vi "writeCounterMasterBatch.vi"(8 "ROI Parameters":T1, 9 "Drop Time (ms)":dbl, 10 "Scan name":string, 11 "file (use dialog)":path) -> ()   [LabVIEW 2015]
uses:
  Controls/ScanParameters/ROI_set.ctl
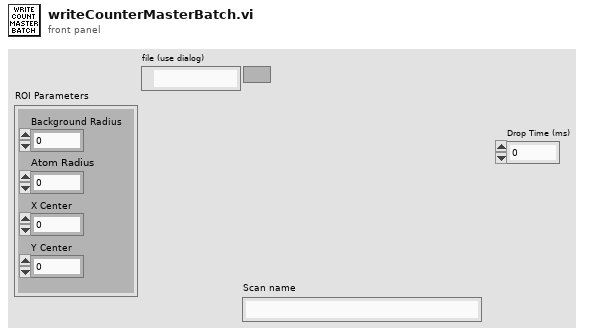
[diagram p1: front panel]
types:
  T1 = typedef "ROI_set.ctl" = cluster{"Background Radius":dbl, "Atom Radius":dbl, "X Center":dbl, "Y Center":dbl}
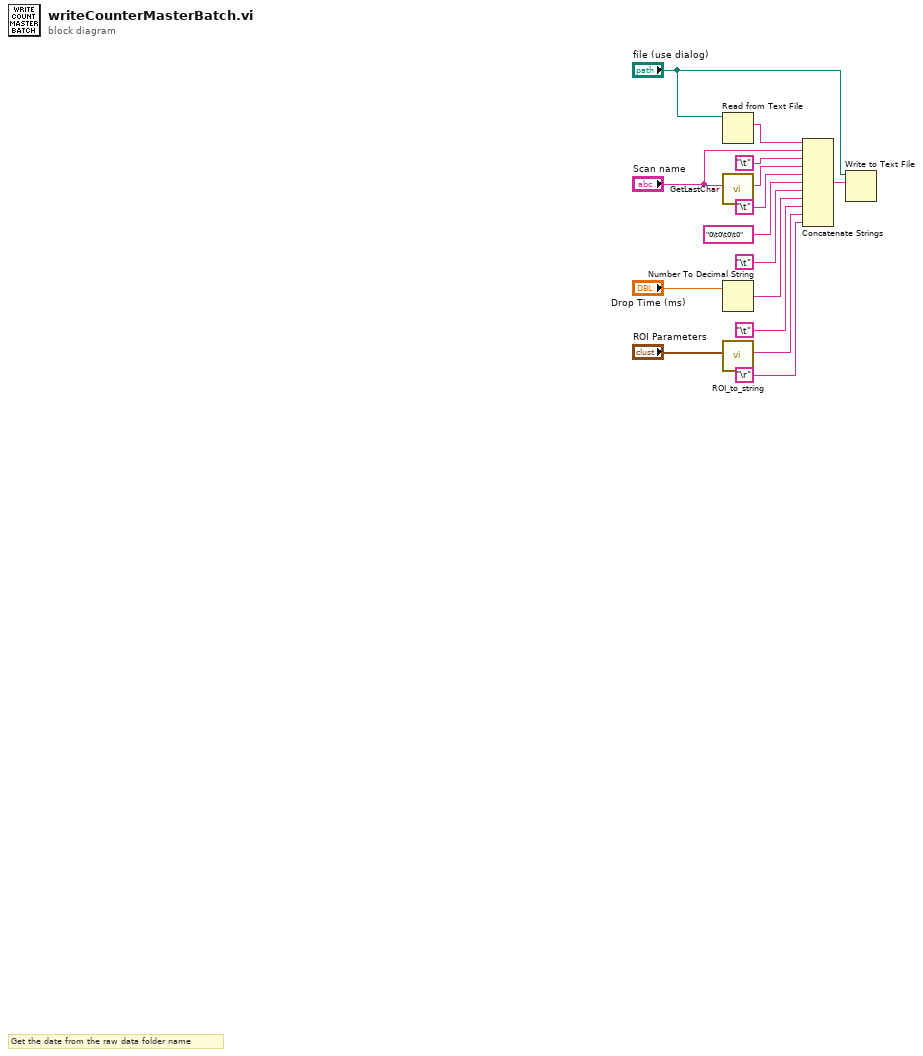
[diagram p0: block diagram]
diagram:
  # "Get the date from the raw data folder name"
  n1 = Read from Text File(file (use dialog)="file (use dialog)") -> (text=w11:string)  [unwired: 3 in, 3 out]
  n2 = call "GetLastChar.vi"("String"="Scan name") -> ("String 2"=w6:string)  [unwired: 10 in]
  n3 = Number To Decimal String(number="Drop Time (ms)") -> (decimal integer string=w12:string)  [unwired: 1 in]
  n4 = call "ROI_to_string.vi"("ROI Parameters"="ROI Parameters") -> ("String"=w14:string)  [unwired: 10 in]
  n5 = Concatenate Strings(w11, "Scan name", "\t", w6, "\t", "0\t0\t0\t0" ("string"), "\t", w12, "\t", w14, "\r") -> (w10:string)
  n6 = Write to Text File(file (use dialog)="file (use dialog)", text=w10) -> ()  [unwired: 2 in, 3 out]
